vi "String to Complex.vi"(11 "string":string) -> (3 "complex number":cdb)   [LabVIEW 2013, in "GOLPI library.lvlib"]
doc: "Converts string with complex number into complex double format. VI suppose complex parts are in %e format and are separated by ' + ' or ' - ' (with spaces)."
uses:
  GOLPI library.lvlib
  <vilib>/regexp/Match Regular Expression.xnode
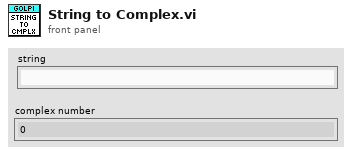
[diagram p1: front panel]
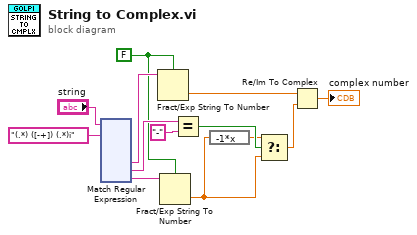
[diagram p0: block diagram]
diagram:
  w5 = FALSE ("use system decimal point (T)")
  n1 = xnode "Match Regular Expression"("input string"="string", "regular expression"="(.*) ([-+]) (.*)i") -> ("submatch 1"=w8:string, "submatch 2"=w10:string, "submatch 3"=w9:string)  [unwired: 4 in, 5 out]
  n2 = Fract/Exp String To Number(use system decimal point (T)=w5, string=w8) -> (number=w3:dbl)  [unwired: 2 in, 1 out]
  n3 = Fract/Exp String To Number(use system decimal point (T)=w5, string=w9) -> (number=w2:dbl)  [unwired: 2 in, 1 out]
  n4 = Equal?(x=w10, y="-") -> (x = y?=w12:bool)
  n5 = expression code="-1*x"(w2) -> (w1:dbl)
  n6 = Select(t=w1, s=w12, f=w2) -> (s? t:f=w13:dbl)
  n7 = Re/Im To Complex(1:w13, 2:w3) -> (0:→"complex number":cdb)
